vi "Stop Core.vi"(10 "final error code":i32, 11 "Console in":refnum<class "Console.lvclass">) -> (3 "Console out":refnum<class "Console.lvclass">)   [LabVIEW 2015, in "EditPanel API.lvlib" / "Console.lvclass"]
doc: "(<B>Filename</B>: Actor Framework.lvlib:Actor.lvclass:Stop Core.vi)\n\nDefines what the actor does before it stops. Use the <B>final error code</B> input to determine whether the actor shut down in response to an error.\n\nBy default, this method does nothing. A descendant class may override it to define behavior, such as shutting down any processes the actor initiated in its override of the Actor Core method."
uses:
  Console.lvclass
  Console.lvclass/Console.ctl
  Console Reply/Console Reply/Console Reply.lvclass/Console Reply.ctl
  <vilib>/ActorFramework/Actor/Actor.lvclass
  Console Reply/Console Reply/Console Reply.lvclass
  EditPanel_class/EditPanel API.lvclass
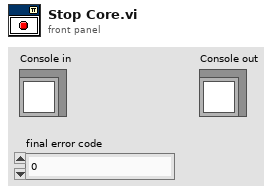
[diagram p1: front panel]
types:
  T1 = enum16{"Attach", "Detach", "Flush", "Update", "Get"}
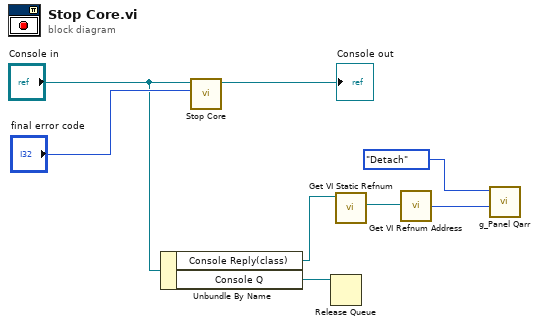
[diagram p0: block diagram]
diagram:
  n1 = Unbundle By Name("Console in") -> ("Console Reply(class)"=w4:refnum<class "Console Reply.lvclass">, "Console Q"=w5:refnum<queue>)
  n2 = call-parent "Stop Core.vi"("final error code"="final error code", "Actor in"="Console in") -> ("Actor out"=→"Console out":refnum<class "Console.lvclass">)  [unwired: 9 in]
  n3 = Release Queue(queue=w5) -> ()  [unwired: 2 in, 3 out]
  n4 = call "Get VI Static Refnum.vi"("Console Reply in"=w4) -> ("VI Static Refnum"=w3:refnum<vi>)  [unwired: 8 in, 2 out]
  n5 = call "Get VI Refnum Address.vi"("VI Refnum"=w3) -> ("Get Ref Address"=w2:u16)
  n6 = call "g_Panel Qarr.vi"("VI Address"=w2, "Operation"=T1."Detach") -> ()  [unwired: 9 in, 1 out]
